vi "Configure RemIO Module.vi"(8 "error in (no error)":errorcluster, 9 "Slave Ref In":refnum<k21>, 10 "11175 in":refnum<class "11175.lvclass">, 11 "Node Ptr In":T1 format="%.0x") -> (0 "error out":errorcluster, 1 "Slave Ref Out":refnum<k21>, 2 "11175 out":refnum<class "11175.lvclass">, 3 "Node Ptr Out":T1 format="%.0x")   [LabVIEW 2016, in "Modules.lvlib" / "11175.lvclass"]
uses:
  11175.lvclass
  <vilib>/NI Veristand/Custom Device API/Custom Device Item Ref.ctl
  11175.lvclass/11175.ctl
  <vilib>/Utility/error.llb/Error Cluster From Error Code.vi
  <vilib>/indcomecat/Remote IO/internal/_Configure REM-11175.vi
  <vilib>/ErrorRing/Error Ring.xnode
  <vilib>/indcomecat/Remote IO/NI ECAT Remote IO.lvlib
  <vilib>/NI Veristand/Custom Device API/Custom Device API.lvlib
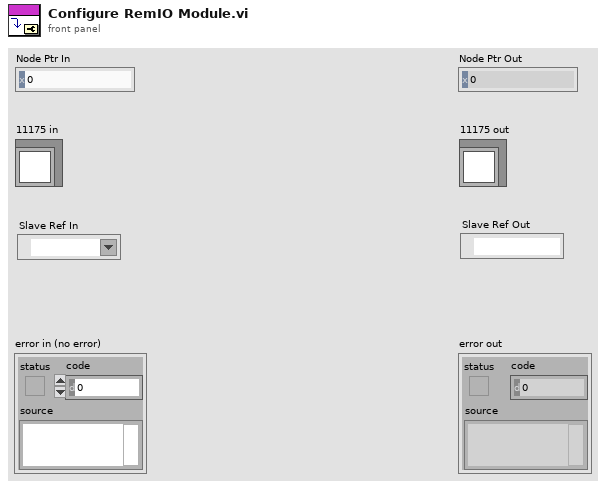
[diagram p1: front panel]
types:
  T1 = typedef "Custom Device API.lvlib/Custom Device Item Ref.ctl" = u64
  T2 = typedef "NI ECAT Remote IO.lvlib/subsititute value on error.ctl" = u8
  T3 = typedef "NI ECAT Remote IO.lvlib/report supply message.ctl" = u8
  T4 = cluster{"substitute value on error":T2, "report \"actuator supply not\npresent\" message?":T3}
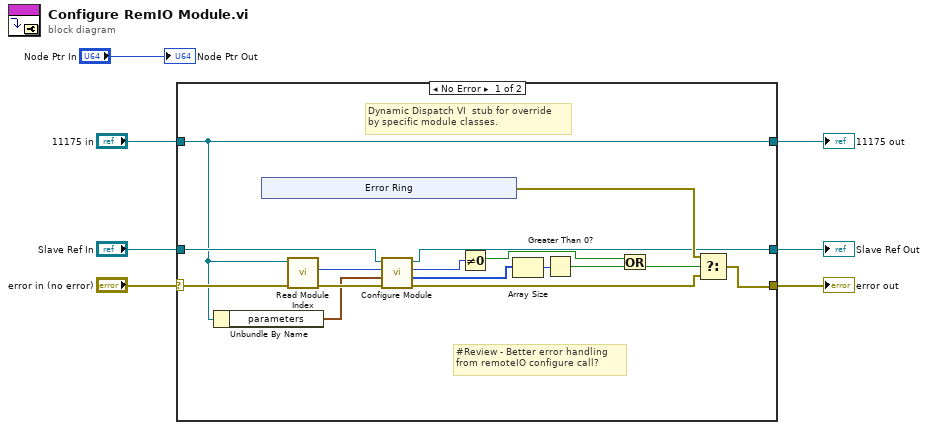
[diagram p0: block diagram]
diagram:
  n1 = case shown="No Error" "error in (no error)" {
    selector: "error in (no error)" -> [w19 w31]
    tunnel: [w20 w31] -> w2
    tunnel: [w13 w30] -> w4
    tunnel: "11175 in" -> [w13 w30]
    tunnel: [w15 w29] -> w3
    tunnel: "Slave Ref In" -> [w16 w29]
    frame No Error {
      # "#Review - Better error handling\nfrom remoteIO configure call?"
      # "Dynamic Dispatch VI  stub for override\nby specific module classes."
      n2 = Unbundle By Name(w13) -> ("parameters"=w12:T4)
      n3 = xnode "Error Ring"() -> ("error out"=w21:errorcluster)
      n4 = call-dynamic "Read Module Index.vi"("error in (no error)"=w19, "RemIO Module in"=w13) -> ("error out"=w18:errorcluster, "Module Index"=w14:u8)  [unwired: 7 in, 1 out]
      n5 = call-poly <vilib>:"Configure Module.vi"("error in (no error)"=w18, "parameters"=w12, "module slot index"=w14, "slave reference in"=w16) -> ("error out"=w17:errorcluster, "negative confirmation"=w11:u8[], "SDO abort code"=w10:u32, "slave reference out"=w15:refnum<k21>)  [unwired: 4 in]
      n6 = Not Equal To 0?(x=w10) -> (x != 0?=w8:bool)
      n7 = Array Size(array=w11) -> (size(s)=w23:i32)
      n8 = Greater Than 0?(x=w23) -> (x > 0?=w22:bool)
      n9 = Or(x=w8, y=w22) -> (x .or. y?=w9:bool)
      n10 = Select(t=w21, s=w9, f=w17) -> (s? t:f=w20:errorcluster)
    }
    frame Error {
    }
  }
  "error out" <- w2
  "11175 out" <- w4
  "Slave Ref Out" <- w3
  "Node Ptr Out" <- "Node Ptr In"
